vi "test.vi"() -> ()   [LabVIEW 2017]
panel:
  out "Boolean 3":bool
  in  "Boolean 2":bool
  in  "Boolean":bool=TRUE
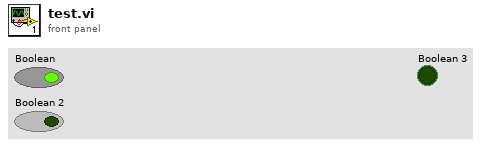
[diagram p1: front panel]
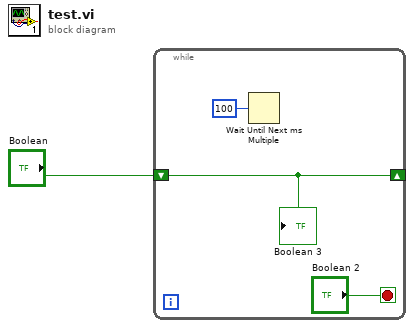
[diagram p0: block diagram]
diagram:
  n1 = while {
    shift-right: [w4] -> _
    shift-left: "Boolean" -> [w4]
    stop <- "Boolean 2" stop-if-true
    n2 = Wait Until Next ms Multiple(millisecond multiple=u32 100 ("milliseconds to wait")) -> ()  [unwired: 1 out]
    "Boolean 3" <- w4
  }
